vi "静态调用的后台任务主调VI.vi"() -> ()   [LabVIEW 2013]
panel:
  out "采集温度":dbl
  out "采集速度":dbl
  in  "停止":bool
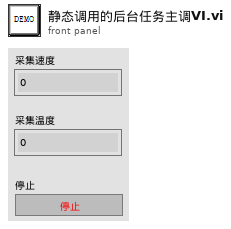
[diagram p1: front panel]
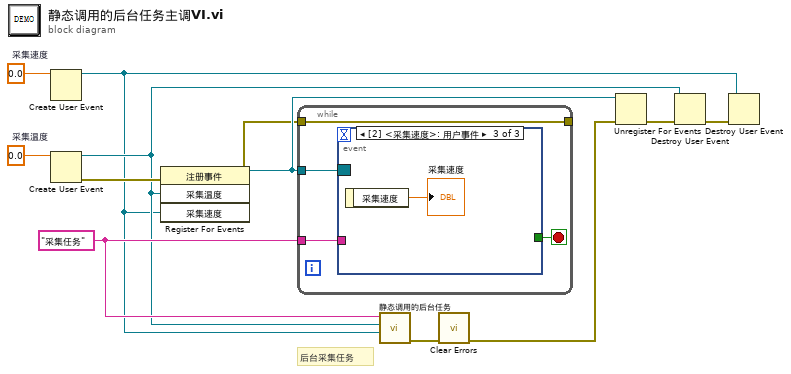
[diagram p0: block diagram]
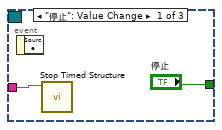
[diagram p2: hidden frame]
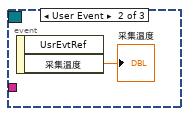
[diagram p3: hidden frame]
diagram:
  w4 = "采集任务" ("结构名称")
  w10 = 0.0  # 采集速度
  w12 = 0.0  # 采集温度
  # "后台采集任务"
  n1 = Create User Event(user event datatype=w10) -> (user event=w2:refnum<user-event>)  [unwired: 1 in, 1 out]
  n2 = Create User Event(user event datatype=w12) -> (user event=w3:refnum<user-event>, error out=w11:errorcluster)  [unwired: 1 in]
  n3 = register-events(error in=w11, w3, w2) -> (reference out=w8:refnum<event-registration>, error out=w6:errorcluster)  [unwired: 1 in]
  n4 = while {
    tunnel: w8 -> [w15]
    tunnel: w4 -> [w14]
    tunnel: w6 -> [w13]
    tunnel: [w13] -> _
    stop <- w16 stop-if-true
    n5 = event shown="[2] <采集速度>: 用户事件" {
      selector: w15 -> [_ _ _]
      dyn-events: _ -> [_ _ _]
      timeout: _ -> [_ _ _]
      tunnel: ["停止" _ _] -> w16
      tunnel: w14 -> [w17 _ _]
      event "停止": Value Change {
        n6 = event-data() -> ()  [unwired: 1 in, 1 out]
        n7 = call <vilib>:"Stop Timed Structure.vi"("name"=w17) -> ()  [unwired: 10 in, 1 out]
      }
      event User Event {
        n8 = event-data() -> ("采集温度"=→"采集温度":dbl)  [unwired: 1 in, 1 out]
      }
      event User Event {
        n9 = event-data() -> ("采集速度"=→"采集速度":dbl)  [unwired: 1 in]
      }
    }
  }
  n10 = call "静态调用的后台任务.vi"("采集速度"=w2, "采集温度"=w3, "结构名称"=w4) -> ("错误输出"=w1:errorcluster)  [unwired: 8 in]
  n11 = call <vilib>:"Clear Errors.vi"("error in (no error)"=w1) -> ("error out"=w5:errorcluster)  [unwired: 6 in]
  n12 = Unregister For Events(event registration refnum=w8, error in=w5) -> (error out=w9:errorcluster)
  n13 = Destroy User Event(user event=w3, error in=w9) -> (error out=w7:errorcluster)
  n14 = Destroy User Event(user event=w2, error in=w7) -> ()  [unwired: 1 out]
